vi "pf_Get_Camera_Property_Mode.vi"(8 "error in (no error)":errorcluster, 10 "Property Name":string, 11 "IMAQ Session in":refnum<k11>) -> (0 "error out":errorcluster, 1 "Mode value":string, 2 "Property Name out":string, 3 "IMAQ Session out":refnum<k11>)   [LabVIEW 2025, in "Photonfocus_Toolkit.lvlib"]
doc: "Gets the value of a Mode type property."
uses:
  Photonfocus_Toolkit.lvlib
  _Private/Controls/pf_Camera_ctrl_mngr_action.ctl
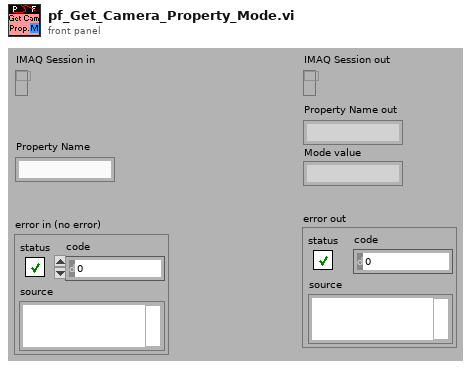
[diagram p1: front panel]
types:
  T1 = typedef "Photonfocus_Toolkit.lvlib/pf_Camera_ctrl_mngr_action.ctl" = enum16{"Create", "Destroy", "Set", "Get"}
  T2 = typedef "Photonfocus_Toolkit.lvlib/pf_Camera_Control.ctl" = cluster{"Port Name":string, "Port Number":i32, "IMAQ Session":refnum<k11>, "PeakDetector_Mode":T3, "Window.W":u32, "Window.H":u32}
  T3 = typedef "Photonfocus_Toolkit.lvlib/pf_PeakDetector_Mode.ctl" = enum16{"Undefined", "2D only", "2D and 3D", "3D only"}
  T4 = typedef "Photonfocus_Toolkit.lvlib/pf_Property_Data_Info.ctl" = cluster{"Type":T5, "Min":string, "Max":string, "MODE Values":string[]}
  T5 = typedef "Photonfocus_Toolkit.lvlib/pf_Property_Type.ctl" = enum16{"Undefined", "PF_ROOT", "PF_INT", "PF_FLOAT", "PF_BOOL", "PF_MODE", "PF_REGISTER", "PF_STRING", "PF_BUFFER", "PF_STRUCT", "PF_ARRAY", "PF_COMMAND", "PF_EVENT"}
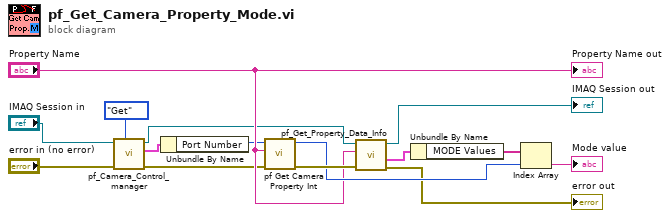
[diagram p0: block diagram]
diagram:
  n1 = call "pf_Camera_Control_manager.vi"("Action"=pf_Camera_ctrl_mngr_action."Get", "error in (no error)"="error in (no error)", "IMAQ Session in"="IMAQ Session in") -> ("error out"=w7:errorcluster, "Camera Control out"=w2:T2, "IMAQ Session out"=w4:refnum<k11>)  [unwired: 1 in, 5 out]
  n2 = Unbundle By Name(w2) -> ("Port Number"=w1:i32)
  n3 = call "pf Get Camera Property Int.vi"("error in (no error)"=w7, "pProperty"="Property Name", "iPort"=w1) -> ("error out"=w15:errorcluster, "function return"=w12:i32)  [unwired: 7 out]
  n4 = call "pf_Get_Property_Data_Info.vi"("error in (no error)"=w15, "Property Name"="Property Name", "IMAQ Session in"=w4) -> ("error out"=→"error out":errorcluster, "Property Data Info"=w9:T4, "IMAQ Session out"=→"IMAQ Session out":refnum<k11>)  [unwired: 6 out]
  n5 = Unbundle By Name(w9) -> ("MODE Values"=w13:string[])
  n6 = Index Array(array=w13, index=w12) -> (element=→"Mode value":string)
  "Property Name out" <- "Property Name"
